vi "ERD Read Pass Fail Test.vi"(0 "GEA2 Reference In":refnum<k24>, 11 "Error In":errorcluster) -> (4 "GEA2 Reference Out":refnum<k24>, 6 "Pass/Fail?":bool, 15 "Error Out":errorcluster)   [LabVIEW 2016, in "2015 VA Washer.lvlib"]
uses:
  Projects/2015 VA Washer.lvlib
  C:/Automation/DLLs/PC Dot Net/GeaCommunication.dll
  Common/LabVIEW GEA2 Toolkit/LabVIEW_GEA2_Toolkit.lvlibp/type defs/ERD Read Data In.ctl
  Common/LabVIEW GEA2 Toolkit/LabVIEW_GEA2_Toolkit.lvlibp/type defs/Data Type.ctl
  Common/LabVIEW GEA2 Toolkit/LabVIEW_GEA2_Toolkit.lvlibp/type defs/Source_Destination.ctl
  Common/LabVIEW GEA2 Toolkit/LabVIEW_GEA2_Toolkit.lvlibp
panel:
  out "Report Text":string
  in  "Expected String":string
  in  "GEA Inputs":T1 {"Destination" format="%.0x"; "Source" format="%.0x"}
  in  "Read ERD List":T2[](array[typedef])=[{"ERD Number"=65535, "Data Type"=enum."string"}] {"ERD Number" format="%.0x"}
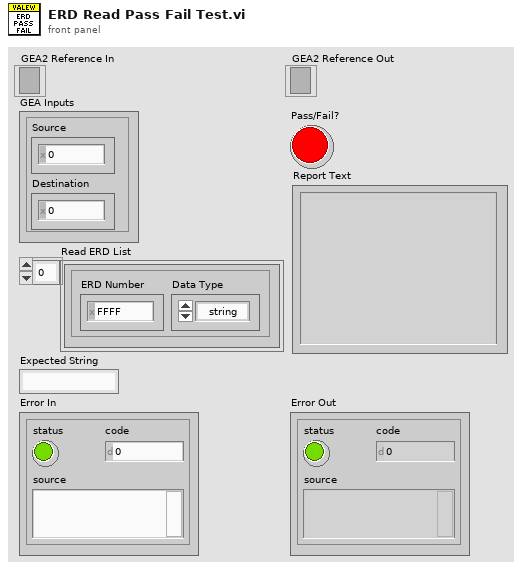
[diagram p1: front panel]
types:
  T1 = typedef "LabVIEW_GEA2_Toolkit.lvlibp/Source_Destination.ctl" = cluster{"Source":u8, "Destination":u8}
  T2 = typedef "LabVIEW_GEA2_Toolkit.lvlibp/ERD Read Data In.ctl" = cluster{"ERD Number":u16, "Data Type":T3}
  T3 = typedef "LabVIEW_GEA2_Toolkit.lvlibp/Data Type.ctl" = enum16{"string", "boolean", "uint8_t", "uint16_t", "uint32_t", "uint64_t", "int8_t", "int16_t", "int32_t", "int64_t"}
  T4 = typedef "LabVIEW_GEA2_Toolkit.lvlibp/ERD Read Data Out.ctl" = cluster{"ERD Number":u16, "Data":string}
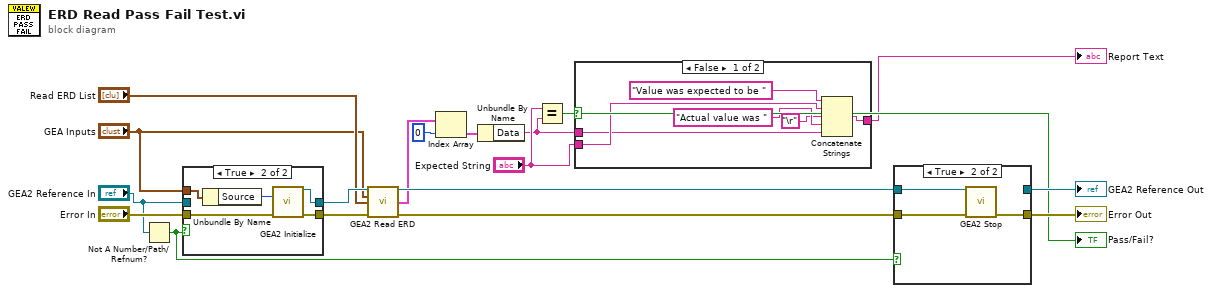
[diagram p0: block diagram]
diagram:
  n1 = Not A Number/Path/Refnum?(number/path/refnum="GEA2 Reference In") -> (NaN/Path/Refnum?=w1:bool)
  n2 = case shown="True" w1 {
    tunnel: "Error In" -> [w19 w25]
    tunnel: [w19 w24] -> w16
    tunnel: "GEA2 Reference In" -> [w20 _]
    tunnel: [w20 w23] -> w14
    tunnel: "GEA Inputs" -> [_ w21]
    frame False {
    }
    frame True {
      n3 = Unbundle By Name(w21) -> ("Source"=w22:u8)
      n4 = call "GEA2 Initialize.vi"("Source Address"=w22, "error in"=w25) -> ("GEA2 Reference Out"=w23:refnum<k24>, "error out"=w24:errorcluster)  [unwired: 11 in, 1 out]
    }
  }
  n5 = call "GEA2 Read ERD.vi"("GEA2 Reference In"=w14, "GEA Inputs"="GEA Inputs", "Read ERD List"="Read ERD List", "Error In"=w16) -> ("GEA2 Reference Out"=w13:refnum<k24>, "ERD Data Out"=w12:T4[], "Error Out"=w15:errorcluster)  [unwired: 8 in, 1 out]
  n6 = Index Array(array=w12, index=0) -> (element=w10:T4)
  n7 = Unbundle By Name(w10) -> ("Data"=w5:string)
  n8 = Equal?(x="Expected String", y=w5) -> (x = y?=w4:bool)
  "Pass/Fail?" <- w4
  n9 = case shown="False" w4 {
    tunnel: [w28 _] -> w3
    tunnel: "Expected String" -> [w27 _]
    tunnel: w5 -> [w26 _]
    frame False {
      n10 = Concatenate Strings("Value was expected to be ", w27, "\r", "Actual value was " ("string"), w26) -> (w28:string)
    }
    frame True {
    }
  }
  "Report Text" <- w3
  n11 = case shown="True" w1 {
    tunnel: [w33 w36] -> w17
    tunnel: w15 -> [w33 w35]
    tunnel: w13 -> [w32 w34]
    tunnel: [w32 _] -> w7
    frame False {
    }
    frame True {
      n12 = call "GEA2 Stop.vi"("GEA2 Reference In"=w34, "Error In"=w35) -> ("Error Out"=w36:errorcluster)  [unwired: 13 in]
    }
  }
  "Error Out" <- w17
  "GEA2 Reference Out" <- w7
